vi "PanelTest1.vi"() -> ()   [LabVIEW 2019]
panel:
  in  "Maxi_visa":refnum<visa-resource-name>
  in  "Measurement Rate (ms)":i32
  out "Channel 6":string
  out "Channel 5":string
  out "Channel 4":string
  out "Channel 3":string
  out "Channel 2":string
  out "Channel 1":string
  # "Pressure Value\n(Torr)"
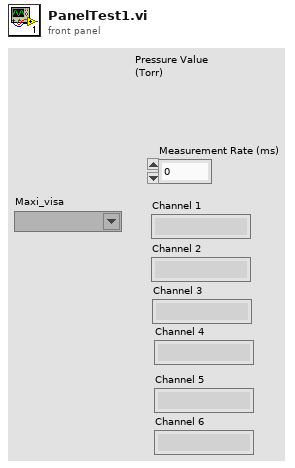
[diagram p1: front panel]
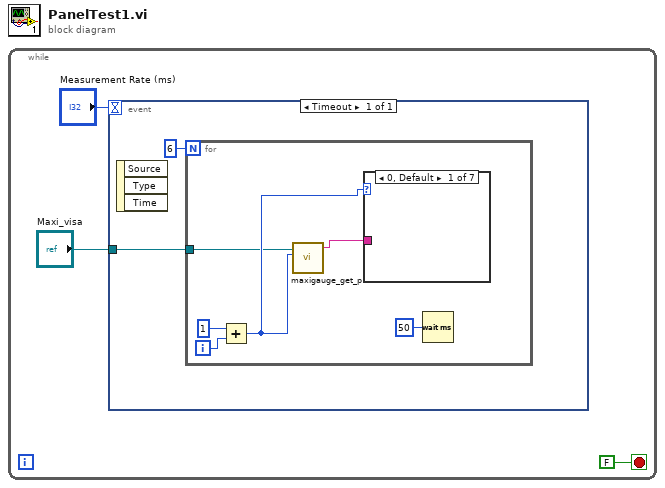
[diagram p0: block diagram]
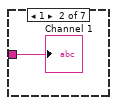
[diagram p2: hidden frame]
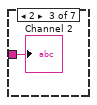
[diagram p3: hidden frame]
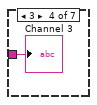
[diagram p4: hidden frame]
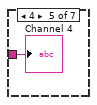
[diagram p5: hidden frame]
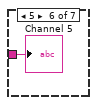
[diagram p6: hidden frame]
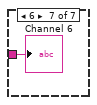
[diagram p7: hidden frame]
diagram:
  n1 = while {
    stop <- FALSE stop-if-true
    n2 = event shown="[0] Timeout" {
      selector: _ -> [_]
      dyn-events: _ -> [_]
      timeout: "Measurement Rate (ms)" -> [_]
      tunnel: "Maxi_visa" -> [w4]
      event Timeout {
        n3 = event-data() -> ()  [unwired: 1 in, 3 out]
        n4 = for {
          N: 6 -> [_]
          tunnel: w4 -> [w6]
          i -> [w11]
          n5 = Add(x=1, y=w11) -> (x+y=w8:i32)
          n6 = call "maxigauge_get_p.vi"(9:w8, "tpg361_visa"=w6) -> ("Pressure (Torr)"=w7:string)  [unwired: 7 in, 1 out]
          n7 = case shown="0, Default" w8 {
            tunnel: w7 -> [_ w12 w13 w14 w15 w16 w17]
            frame 0, Default {
            }
            frame 1 {
              "Channel 1" <- w12
            }
            frame 2 {
              "Channel 2" <- w13
            }
            frame 3 {
              "Channel 3" <- w14
            }
            frame 4 {
              "Channel 4" <- w15
            }
            frame 5 {
              "Channel 5" <- w16
            }
            frame 6 {
              "Channel 6" <- w17
            }
          }
          n8 = Wait (ms)(milliseconds to wait=u32 50) -> ()  [unwired: 1 out]
        }
      }
    }
  }
